vi "Add_Version_Info.vi"(0 "String Array In":string[](array[string]), 2 "All_ERD_Data_Bundled_Brass out":T1) -> (14 "String Array Out":string[](array[string]))   [LabVIEW 2019]
uses:
  type defs/All_Bundled_Data_JL.ctl
  type defs/Version.ctl
  type defs/ERD_Always_Show_JL.ctl
  type defs/CSV_File_String_Arrays.ctl
  type defs/Fault Table Array.ctl
  type defs/Fault_Table_Info.ctl
  type defs/Heat Control.ctl
panel:
  # "Software Version"
  # "Critical Version"
  # "Non-Critical"
  # "Software Version"
  # "Critical Version"
  # "Non-Critical"
  # "XML Crit Ver"
  # "XML Non-Crit"
  # "Build Number"
  # "Build Hash"
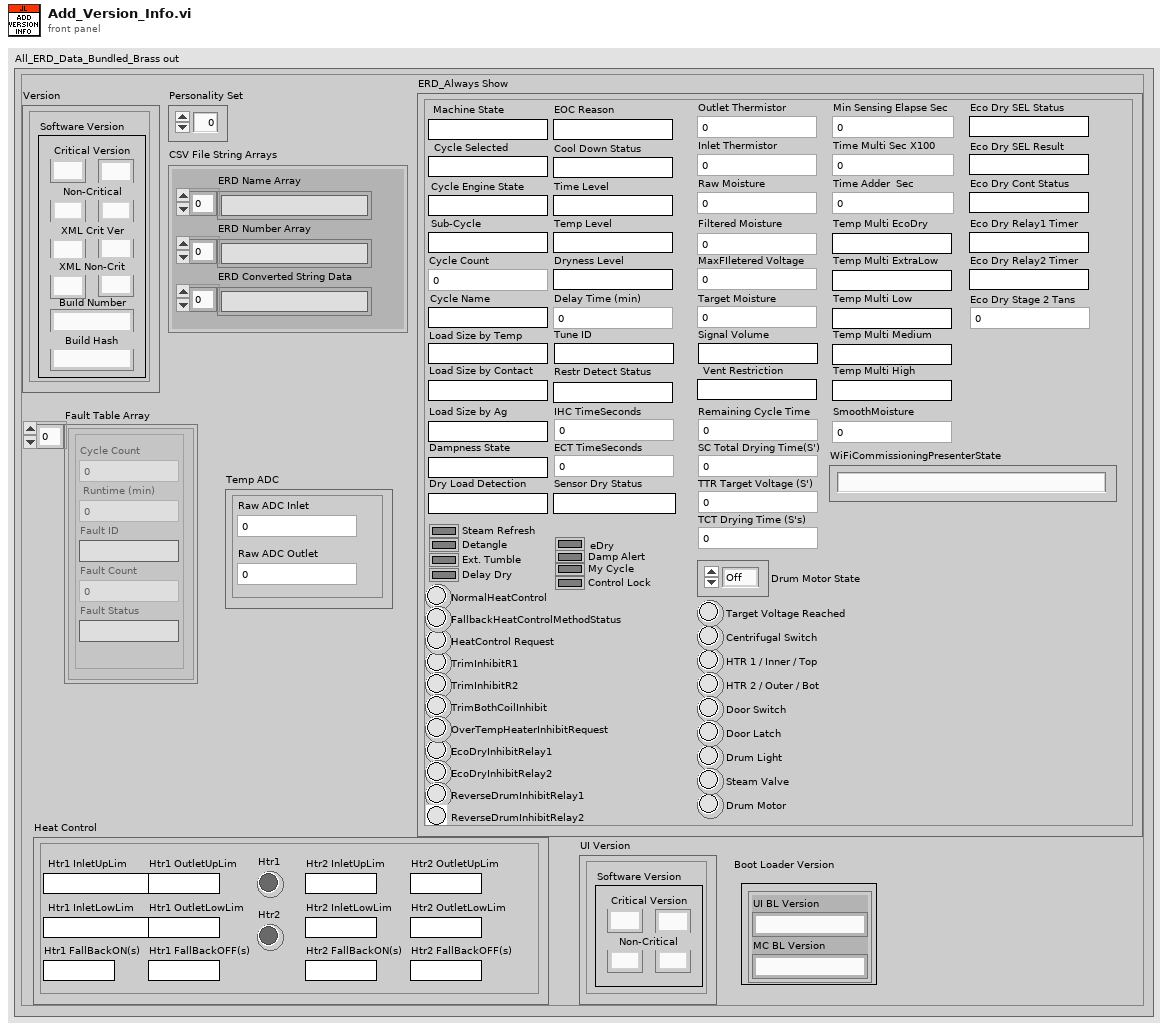
[diagram p1: front panel]
types:
  T1 = typedef "All_Bundled_Data_JL.ctl" = cluster{"Version":T2, "ERD_Always Show":T3, "Personality Set":u8, "CSV File String Arrays":T4, "Fault Table Array ":T5, "Heat Control":T7, "Temp ADC":cluster{"Raw ADC Outlet":u16, "Raw ADC Inlet":u16}, "UI Version":cluster{"Critical Major":string, "Critical Minor":string, "Non-Critical Minor":string, "Non-Critical Major":string}, "Boot Loader Version":cluster{"UI BL Version":string, "MC BL Version":string}}
  T2 = typedef "Version.ctl" = cluster{"Critical Major":string, "Critical Minor":string, "Non-Critical Minor":string, "Non-Critical Major":string, "XML Crit Minor":string, "XMLCrit Major":string, "Build Number":string, "XML Non-crit Minor":string, "Xml Non-crit Major":string, "Build Hash":string}
  T3 = typedef "ERD_Always_Show_JL.ctl" = cluster{"Inlet Thermistor":u16, "Machine State":string, "Filtered Moisture":u16, "Cycle Selected":string, "HTR 1 / Inner / Top":bool, "HTR 2 / Outer / Bot":bool, "Door Switch":bool, "Drum Light":bool, "Cycle Engine State":string, "Centrifugal Switch":bool, "Drum Motor":bool, "Cycle Count":u32, "Ext. Tumble":bool, "eDry":bool, "Temp Level":string, "Dryness Level":string, "Time Level":string, "Delay Time (min)":u16, "Steam Refresh":bool, "Damp Alert":bool, "Sub-Cycle":string, "Outlet Thermistor":u16, "Target Moisture":u16, "Remaining Cycle Time":u32, "Raw Moisture":u16, "Cycle Name":string, "My Cycle":bool, "Delay Dry":bool, "Detangle":bool, "Control Lock":bool, "Steam Valve":bool, "Door Latch":bool, "Signal Volume":string, "Tune ID":string, "Restr Detect Status":string, "Vent Restriction":string, "Load Size by Contact":string, "Load Size by Temp":string, "EOC Reason":string, "Sensor Dry Status":string, "Dampness State":string, "Target Voltage Reached":bool, "TrimInhibitR1":bool, "TrimInhibitR2":bool, "TrimBothCoilInhibit":bool, "NormalHeatControl":bool, "HeatControl Request":bool, "Cool Down Status":string, "EcoDryInhibitRelay1":bool, "EcoDryInhibitRelay2":bool, "ReverseDrumInhibitRelay1":bool, "ReverseDrumInhibitRelay2":bool, "OverTempHeaterInhibitRequest":bool, "FallbackHeatControlMethodStatus":bool, "IHC TimeSeconds":u32, "ECT TimeSeconds ":u32, "SC Total Drying Time(S')":u32, "TTR Target Voltage (S')":u32, "TCT Drying Time (S's)":u32, "Drum Motor State":enum16{"Off", "Cw", "Ccw", "Max"}, "Load Size by Ag":string, "MaxFIletered Voltage":u16, "Dry Load Detection":string, "Min Sensing Elapse Sec":u32, "Time Multi Sec X100":u32, "Time Adder  Sec":u32, "Temp Multi EcoDry":string, "Temp Multi ExtraLow":string, "Temp Multi Low ":string, "Temp Multi Medium":string, "Temp Multi High":string, "SmoothMoisture":u16, "Eco Dry SEL Status":string, "Eco Dry SEL Result":string, "Eco Dry Cont Status":string, "Eco Dry Relay1 Timer":string, "Eco Dry Relay2 Timer ":string, "Eco Dry Stage 2 Tans ":u32, "WiFiCommissioningPresenterState":string}
  T4 = typedef "CSV_File_String_Arrays.ctl" = cluster{"ERD Number Array":string[], "ERD Name Array":string[], "ERD Converted String Data":string[]}
  T5 = typedef "Fault Table Array.ctl" = T6[]
  T6 = typedef "Fault_Table_Info.ctl" = cluster{"Cycle Count":u32, " Runtime (min) ":u32, "Fault Status":string, "Fault ID":string, "Fault Count":u16}
  T7 = typedef "Heat Control.ctl" = cluster{"Htr1 InletLowLim":string, "Htr1 InletUpLim":string, "Htr1 OutletLowLim":string, "Htr1 OutletUpLim":string, "Htr1 FallBackON(s)":string, "Htr1 FallBackOFF(s)":string, "Htr1":bool, "Htr2 InletLowLim":string, "Htr2 InletUpLim":string, "Htr2 OutletLowLim":string, "Htr2 OutletUpLim":string, "Htr2 FallBackON(s)":string, "Htr2 FallBackOFF(s)":string, "Htr2":bool}
  T8 = cluster{"UI BL Version":string, "MC BL Version":string}
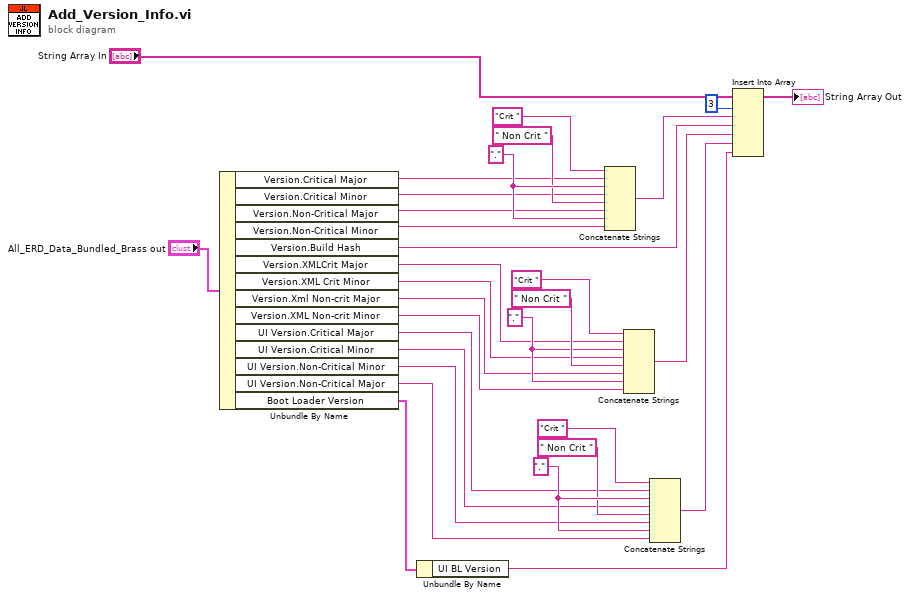
[diagram p0: block diagram]
diagram:
  w10 = "." ("element")
  w16 = "." ("element")
  w28 = "." ("element")
  n1 = Unbundle By Name("All_ERD_Data_Bundled_Brass out") -> ("Version.Critical Major"=w24:string, "Version.Critical Minor"=w23:string, "Version.Non-Critical Major"=w22:string, "Version.Non-Critical Minor"=w21:string, "Version.Build Hash"=w19:string, "Version.XMLCrit Major"=w15:string, "Version.XML Crit Minor"=w14:string, "Version.Xml Non-crit Major"=w13:string, "Version.XML Non-crit Minor"=w12:string, "UI Version.Critical Major"=w7:string, "UI Version.Critical Minor"=w6:string, "UI Version.Non-Critical Minor"=w5:string, "UI Version.Non-Critical Major"=w4:string, "Boot Loader Version"=w2:T8)
  n2 = Unbundle By Name(w2) -> ("UI BL Version"=w1:string)
  n3 = Concatenate Strings("Crit " ("element"), w24, w28, w23, " Non Crit " ("element"), w22, w28, w21) -> (w20:string)
  n4 = Concatenate Strings("Crit " ("element"), w15, w16, w14, " Non Crit " ("element"), w13, w16, w12) -> (w11:string)
  n5 = Concatenate Strings("Crit " ("element"), w7, w10, w6, " Non Crit " ("element"), w5, w10, w4) -> (w3:string)
  n6 = Insert Into Array(array="String Array In", index=3, new element #1=w20, new element #2=w19, new element #3=w11, new element #4=w3, new element #5=w1) -> (→"String Array Out":string[])
